vi "Start.vi"(8 "error in (no error)":errorcluster, 10 "Builder":refnum<class "Builder.lvclass">) -> (0 "error out":errorcluster, 3 "Simple Build GUI out":refnum<class "Simple Build GUI.lvclass">)   [LabVIEW 2020, in "Builder Tools.lvlib" / "Simple Build GUI.lvclass"]
uses:
  Simple Build GUI.lvclass
  Simple Build GUI.lvclass/Simple Build GUI.ctl
  Builder/Builder.lvclass
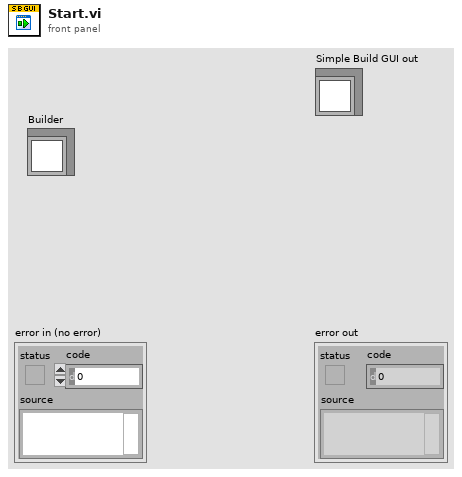
[diagram p1: front panel]
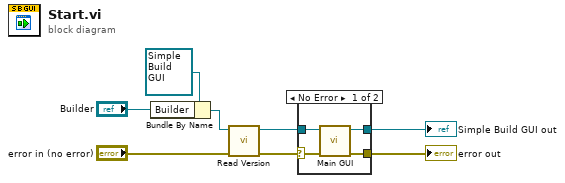
[diagram p0: block diagram]
diagram:
  n1 = Bundle By Name(cluster=refnum<class "Simple Build GUI.lvclass"> refnum ("Simple Build GUI in"), "Builder"="Builder") -> (w4:refnum<class "Simple Build GUI.lvclass">)
  n2 = call "Read Version.vi"("error in (no error)"="error in (no error)", "Simple Build GUI in"=w4) -> ("error out"=w5:errorcluster, "Simple Build GUI out"=w2:refnum<class "Simple Build GUI.lvclass">)  [unwired: 8 in]
  n3 = case shown="No Error" w5 {
    selector: w5 -> [w12 w14]
    tunnel: [w11 w14] -> w3
    tunnel: w2 -> [w10 w13]
    tunnel: [w9 w13] -> w1
    frame No Error {
      n4 = call "Main GUI.vi"("error in (no error)"=w12, "Simple Build GUI in"=w10) -> ("error out"=w11:errorcluster, "Simple Build GUI out"=w9:refnum<class "Simple Build GUI.lvclass">)  [unwired: 8 in]
    }
    frame Error {
    }
  }
  "error out" <- w3
  "Simple Build GUI out" <- w1
